vi "DSF.Engine.Framework.Create.Transfer Groups.vi"(8 "error in (no error)":errorcluster, 10 "Transfer Group Configurations":refnum<class "DSF.Shared.Configuration.Transfer Group.lvclass">[](array[class]), 11 "Framework in":refnum<class "DSF.Engine.Framework.lvclass">) -> (0 "error out":errorcluster, 2 "Transfer Groups":refnum<class "DSF.Engine.Transfer Group.lvclass">[](array[class]), 3 "Framework out":refnum<class "DSF.Engine.Framework.lvclass">)   [LabVIEW 2017, in "DSF.Engine.lvlib" / "DSF.Engine.Framework.lvclass"]
uses:
  DSF.Engine.Framework.lvclass
  Transfer/DSF.Engine.Transfer Group.lvclass
  Shared/Classes/Transfer Group/DSF.Shared.Configuration.Transfer Group.lvclass
  DSF.Engine.Framework.lvclass/DSF.Engine.Framework.ctl
  Cache/DSF.Engine.Memory.Cache.lvclass/DSF.Engine.Memory.Cache.ctl
  Shared/Classes/Transfer Group/DSF.Shared.Configuration.Transfer Group.lvclass/DSF.Shared.Configuration.Transfer Group.ctl
  Timing/DSF.Engine.Timing.lvclass
  Cache/DSF.Engine.Memory.Cache.lvclass
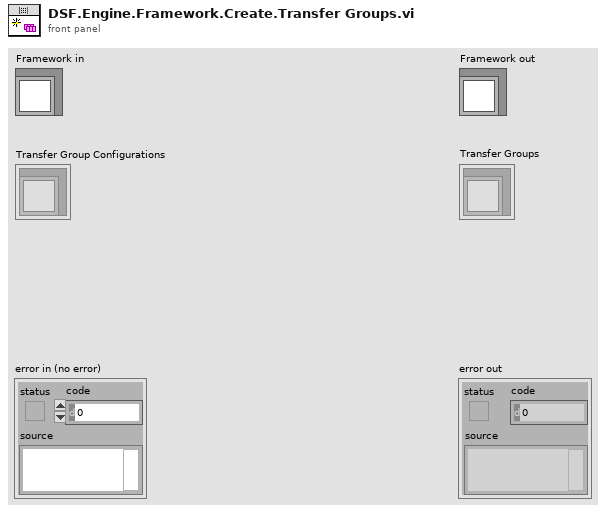
[diagram p1: front panel]
types:
  T1 = typedef "DSF.Shared.lvlib/DSF.Shared.Typedefs.Direction.ctl" = enum8{"Tx", "Rx"}
  T2 = typedef "DSF.Shared.lvlib/DSF.Shared.Typedefs.Cycle Timing Factors.ctl" = cluster{"Priority":u64, "Decimation":u64, "Offset":u64}
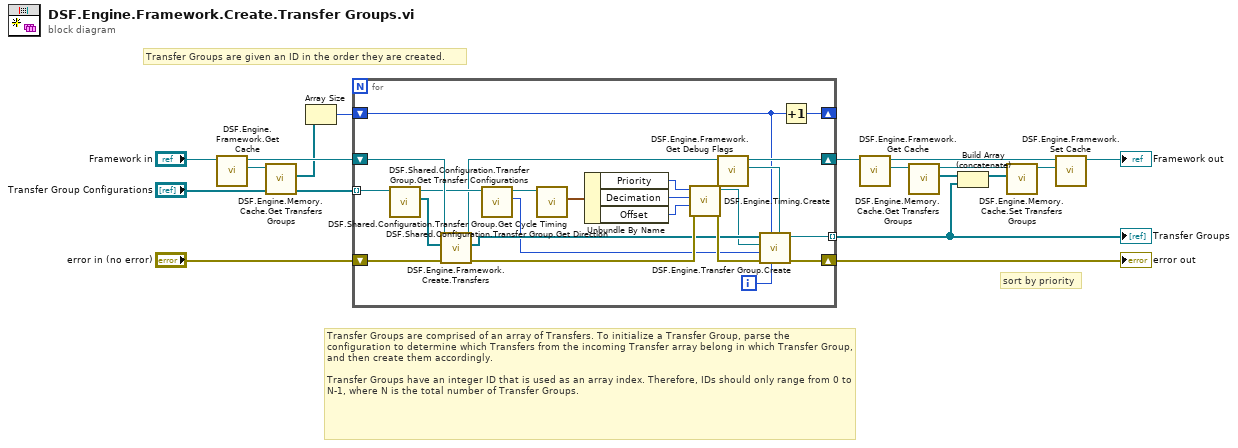
[diagram p0: block diagram]
diagram:
  # "Transfer Groups are given an ID in the order they are created."
  # "sort by priority"
  # "Transfer Groups are comprised of an array of Transfers. To initialize a Transfer Group, parse the configuration to determine which Transfers from the incoming Transfer array belong in which Transfer Group, and then create them accordingly.\n\nTransfer Groups have an integer ID that is used as an array index. Therefore, IDs should only range from 0 to N-1, where N is the total number of Transfer Groups."
  n1 = call "DSF.Engine.Framework.Get Cache.vi"("Framework in"="Framework in") -> ("Cache"=w6:refnum<class "DSF.Engine.Memory.Cache.lvclass">, "Framework out"=w4:refnum<class "DSF.Engine.Framework.lvclass">)  [unwired: 9 in]
  n2 = call "DSF.Engine.Memory.Cache.Get Transfers Groups.vi"("Cache in"=w6) -> ("Transfers Groups"=w3:refnum<class "DSF.Engine.Transfer Group.lvclass">[])  [unwired: 9 in, 1 out]
  n3 = Array Size(array=w3) -> (size(s)=w16:i32)
  n4 = for {
    shift-right: [w40] -> w1
    shift-left: "error in (no error)" -> [w38]
    tunnel: [w18] -> w2 mode=indexing
    shift-right: [w22] -> w8
    shift-left: w4 -> [w25]
    shift-right: [w37] -> _
    shift-left: w16 -> [w20]
    tunnel: "Transfer Group Configurations" -> [w39] mode=indexing
    i -> [w19]
    n5 = call "DSF.Shared.Configuration.Transfer Group.Get Transfer Configurations.vi"("Transfer Group Configuration in"=w39) -> ("Transfer Configurations"=w36:refnum<class "DSF.Shared.Configuration.Transfer.lvclass">[], "Transfer Group Configuration out"=w24:refnum<class "DSF.Shared.Configuration.Transfer Group.lvclass">)  [unwired: 9 in]
    n6 = call "DSF.Engine.Framework.Create.Transfers.vi"("error in (no error)"=w38, "Transfer Configurations"=w36, "Framework in"=w25) -> ("error out"=w33:errorcluster, "Transfers"=w28:refnum<class "DSF.Engine.Transfer.lvclass">[], "Framework out"=w23:refnum<class "DSF.Engine.Framework.lvclass">)  [unwired: 6 in]
    n7 = call "DSF.Shared.Configuration.Transfer Group.Get Direction.vi"("Transfer Group Configuration in"=w24) -> ("direction"=w26:T1, "Transfer Group Configuration out"=w35:refnum<class "DSF.Shared.Configuration.Transfer Group.lvclass">)  [unwired: 9 in]
    n8 = call "DSF.Shared.Configuration.Transfer Group.Get Cycle Timing.vi"("Transfer Group Configuration in"=w35) -> ("cycle timing"=w34:T2)  [unwired: 9 in, 1 out]
    n9 = Unbundle By Name(w34) -> ("Priority"=w29:u64, "Decimation"=w30:u64, "Offset"=w31:u64)
    n10 = call "DSF.Engine.Timing.Create.vi"("error in (no error)"=w33, "Offset"=w31, "Decimation"=w30, "Priority"=w29) -> ("error out"=w32:errorcluster, "Timing"=w27:refnum<class "DSF.Engine.Timing.lvclass">)  [unwired: 6 in]
    n11 = call "DSF.Engine.Framework.Get Debug Flags.vi"("Framework in"=w23) -> ("Debug Flags"=w21:refnum<class "DSF.Engine.Debug Flags.lvclass">, "Framework out"=w22:refnum<class "DSF.Engine.Framework.lvclass">)  [unwired: 9 in]
    n12 = call "DSF.Engine.Transfer Group.Create.vi"("Debug Flags"=w21, "transceiver id"=w19, "framework id"=w20, "error in (no error)"=w32, "Direction"=w26, "Timing"=w27, "Transfers"=w28) -> ("error out"=w40:errorcluster, "Transfer Group out"=w18:refnum<class "DSF.Engine.Transfer Group.lvclass">)  [unwired: 3 in]
    n13 = Increment(x=w20) -> (x+1=w37:i32)
  }
  "error out" <- w1
  "Transfer Groups" <- w2
  n14 = call "DSF.Engine.Framework.Get Cache.vi"("Framework in"=w8) -> ("Cache"=w13:refnum<class "DSF.Engine.Memory.Cache.lvclass">, "Framework out"=w14:refnum<class "DSF.Engine.Framework.lvclass">)  [unwired: 9 in]
  n15 = call "DSF.Engine.Memory.Cache.Get Transfers Groups.vi"("Cache in"=w13) -> ("Transfers Groups"=w10:refnum<class "DSF.Engine.Transfer Group.lvclass">[], "Cache out"=w11:refnum<class "DSF.Engine.Memory.Cache.lvclass">)  [unwired: 9 in]
  n16 = Build Array (concatenate)(w10, w2) -> (w9:refnum<class "DSF.Engine.Transfer Group.lvclass">[])
  n17 = call "DSF.Engine.Memory.Cache.Set Transfers Groups.vi"("Transfers Groups"=w9, "Cache in"=w11) -> ("Cache out"=w12:refnum<class "DSF.Engine.Memory.Cache.lvclass">)  [unwired: 9 in]
  n18 = call "DSF.Engine.Framework.Set Cache.vi"("Cache"=w12, "Framework in"=w14) -> ("Framework out"=→"Framework out":refnum<class "DSF.Engine.Framework.lvclass">)  [unwired: 9 in]
